vi "generateSQL.vi"(0 "input cluster":T1) -> (1 "SQL command (mote)":string, 2 "SQL command (plc)":string, 3 "SQL command (counter and manual)":string)   [LabVIEW 2011]
panel:
  out "plc":string[](array[string])
  out "mote":string[](array[string])
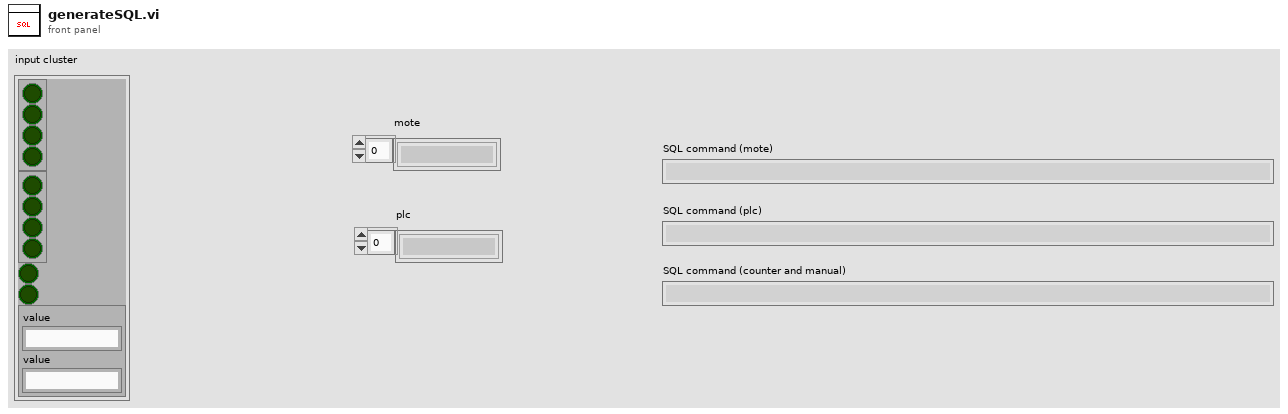
[diagram p1: front panel]
types:
  T1 = cluster{cluster{bool, bool, bool, bool}, cluster{bool, bool, bool, bool}, bool, bool, cluster{"value":string, "value":string}}
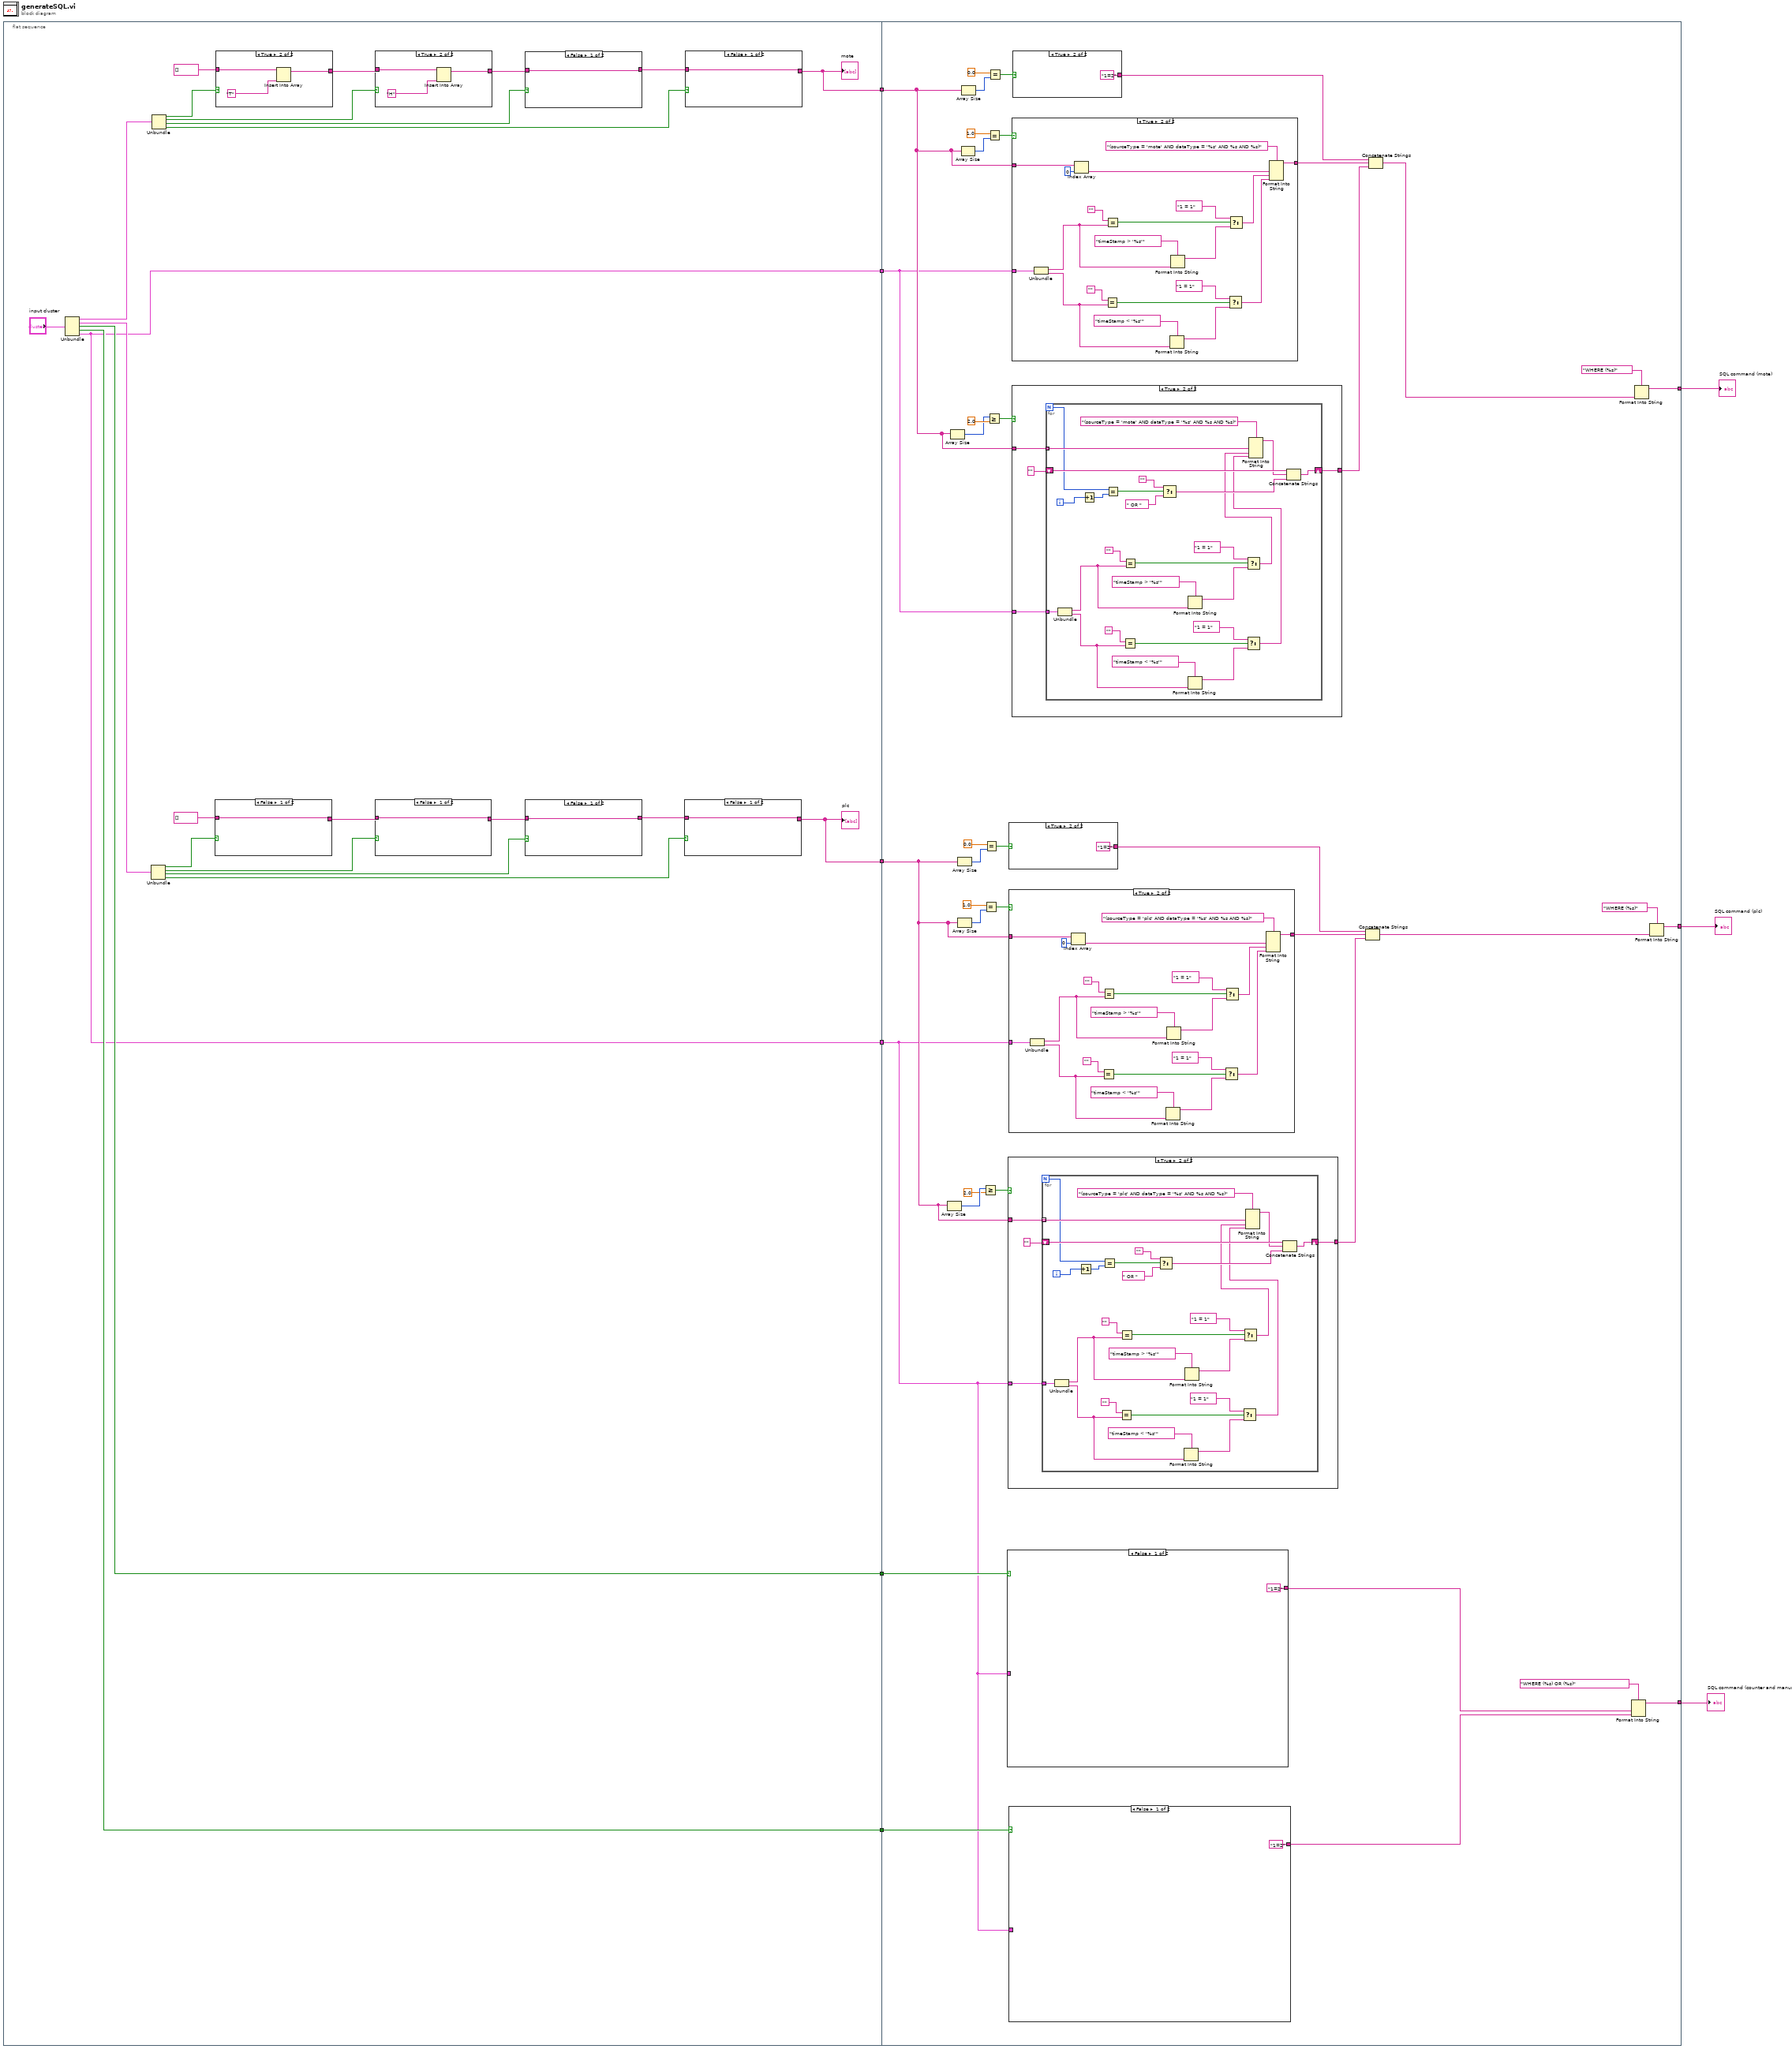
[diagram p0: block diagram]
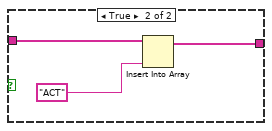
[diagram p2: hidden frame]
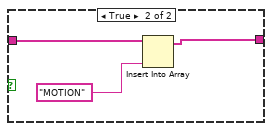
[diagram p3: hidden frame]
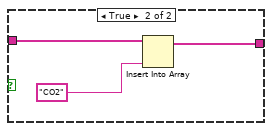
[diagram p4: hidden frame]
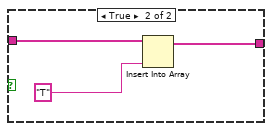
[diagram p5: hidden frame]
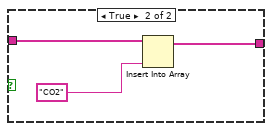
[diagram p6: hidden frame]
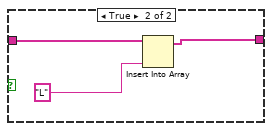
[diagram p7: hidden frame]
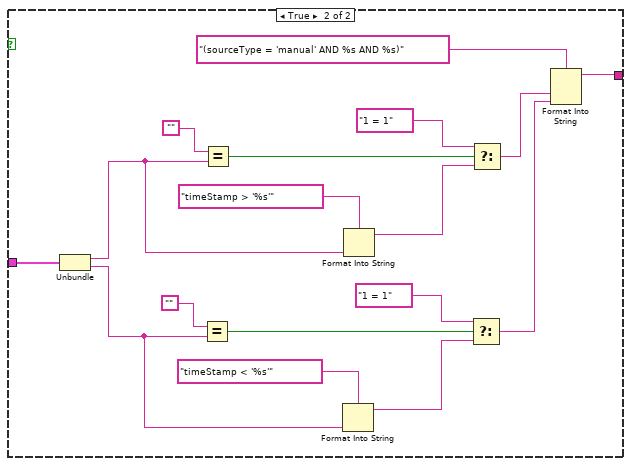
[diagram p10: hidden frame]
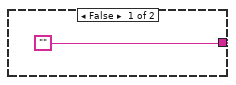
[diagram p11: hidden frame]
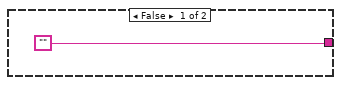
[diagram p12: hidden frame]
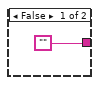
[diagram p13: hidden frame]
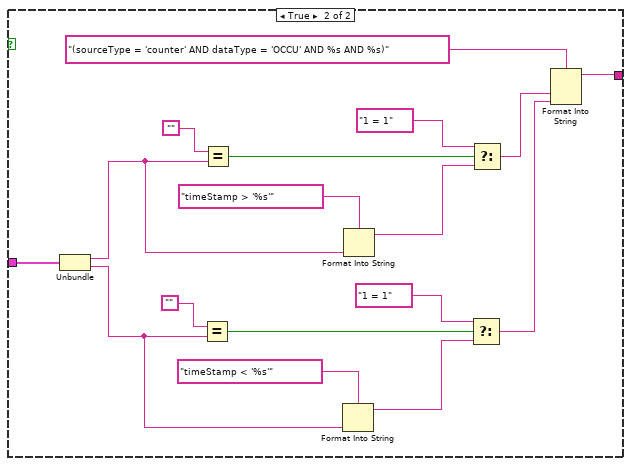
[diagram p14: hidden frame]
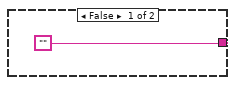
[diagram p15: hidden frame]
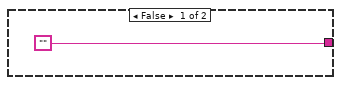
[diagram p16: hidden frame]
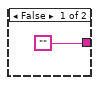
[diagram p17: hidden frame]
diagram:
  n1 = flat-sequence {
    tunnel: [w14] -> w9
    tunnel: [w13] -> w7
    tunnel: [w12] -> w6
    tunnel: [w10] -> w5
    tunnel: [w11] -> w4
    tunnel: [w10] -> w3
    tunnel: w9 -> [w93]
    tunnel: [w90] -> w8
    tunnel: w7 -> [w89]
    tunnel: w6 -> [w74]
    tunnel: w5 -> [w88]
    tunnel: w4 -> [w75]
    tunnel: w3 -> [w73]
    tunnel: [w69] -> w2
    tunnel: [w68] -> w1
    frame #0 {
      n2 = Unbundle("input cluster") -> (w32:cluster{bool, bool, bool, bool}, w31:cluster{bool, bool, bool, bool}, w13:bool, w12:bool, w10:cluster{"value":string, "value":string})
      n3 = Unbundle(w31) -> (w18:bool, w17:bool, w16:bool, w15:bool)
      n4 = Unbundle(w32) -> (w30:bool, w28:bool, w26:bool, w25:bool)
      n5 = case shown="False" w18 {
        tunnel: string[] [] -> [w46 w48]
        tunnel: [w46 w47] -> w20
        frame False {
        }
        frame True {
          n6 = Insert Into Array(array=w48, new element="T") -> (w47:string[])  [unwired: 1 in]
        }
      }
      n7 = case shown="True" w30 {
        tunnel: string[] [] -> [w62 w64]
        tunnel: [w62 w63] -> w27
        frame False {
        }
        frame True {
          n8 = Insert Into Array(array=w64, new element="T") -> (w63:string[])  [unwired: 1 in]
        }
      }
      n9 = case shown="False" w17 {
        tunnel: w20 -> [w42 w44]
        tunnel: [w42 w43] -> w21
        frame False {
        }
        frame True {
          n10 = Insert Into Array(array=w44, new element="CO2") -> (w43:string[])  [unwired: 1 in]
        }
      }
      n11 = case shown="True" w28 {
        tunnel: w27 -> [w58 w60]
        tunnel: [w58 w59] -> w24
        frame False {
        }
        frame True {
          n12 = Insert Into Array(array=w60, new element="H") -> (w59:string[])  [unwired: 1 in]
        }
      }
      n13 = case shown="False" w16 {
        tunnel: w21 -> [w38 w40]
        tunnel: [w38 w39] -> w22
        frame False {
        }
        frame True {
          n14 = Insert Into Array(array=w40, new element="MOTION") -> (w39:string[])  [unwired: 1 in]
        }
      }
      n15 = case shown="False" w26 {
        tunnel: w24 -> [w54 w56]
        tunnel: [w54 w55] -> w23
        frame False {
        }
        frame True {
          n16 = Insert Into Array(array=w56, new element="L") -> (w55:string[])  [unwired: 1 in]
        }
      }
      n17 = case shown="False" w15 {
        tunnel: w22 -> [w34 w36]
        tunnel: [w34 w35] -> w11
        frame False {
        }
        frame True {
          n18 = Insert Into Array(array=w36, new element="ACT") -> (w35:string[])  [unwired: 1 in]
        }
      }
      "plc" <- w11
      n19 = case shown="False" w25 {
        tunnel: w23 -> [w50 w52]
        tunnel: [w50 w51] -> w14
        frame False {
        }
        frame True {
          n20 = Insert Into Array(array=w52, new element="CO2") -> (w51:string[])  [unwired: 1 in]
        }
      }
      "mote" <- w14
    }
    frame #1 {
      n21 = Array Size(array=w75) -> (size(s)=w84:i32)
      n22 = Array Size(array=w93) -> (size(s)=w97:i32)
      n23 = Array Size(array=w75) -> (size(s)=w80:i32)
      n24 = Array Size(array=w75) -> (size(s)=w77:i32)
      n25 = Array Size(array=w93) -> (size(s)=w101:i32)
      n26 = Array Size(array=w93) -> (size(s)=w104:i32)
      n27 = Greater Or Equal?(x=w84, y=2.0) -> (x >= y?=w82:bool)
      n28 = Equal?(x=1.0, y=w80) -> (x = y?=w79:bool)
      n29 = Equal?(x=0.0, y=w77) -> (x = y?=w78:bool)
      n30 = Greater Or Equal?(x=w97, y=2.0) -> (x >= y?=w99:bool)
      n31 = Equal?(x=1.0, y=w101) -> (x = y?=w102:bool)
      n32 = Equal?(x=0.0, y=w104) -> (x = y?=w103:bool)
      n33 = case shown="False" w89 {
        tunnel: ["1=2" w180] -> w67
        tunnel: w73 -> [_ w184]
        frame False {
        }
        frame True {
          n34 = Unbundle(w184) -> ("value"=w192:string, "value"=w185:string)
          n35 = Equal?(x="", y=w185) -> (x = y?=w187:bool)
          n36 = Equal?(x="", y=w192) -> (x = y?=w195:bool)
          n37 = Format Into String(format string="timeStamp < '%s'", w185) -> (resulting string=w189:string)  [unwired: 2 in, 1 out]
          n38 = Format Into String(format string="timeStamp > '%s'", w192) -> (resulting string=w193:string)  [unwired: 2 in, 1 out]
          n39 = Select(t="1 = 1", s=w187, f=w189) -> (s? t:f=w182:string)
          n40 = Select(t="1 = 1", s=w195, f=w193) -> (s? t:f=w183:string)
          n41 = Format Into String(format string="(sourceType = 'counter' AND dataType = 'OCCU' AND %s AND %s)", w183, w182) -> (resulting string=w180:string)  [unwired: 2 in, 1 out]
        }
      }
      n42 = case shown="True" w82 {
        tunnel: w75 -> [_ w126]
        tunnel: ["" w127] -> w87
        tunnel: w73 -> [_ w125]
        frame False {
        }
        frame True {
          n43 = for {
            N -> [w150]
            shift-right: [w152] -> w127
            shift-left: "" -> [w154]
            tunnel: w126 -> [w151] mode=indexing
            tunnel: w125 -> [w129]
            i -> [w148]
            n44 = Unbundle(w129) -> ("value"=w136:string, "value"=w143:string)
            n45 = Increment(x=w148) -> (x+1=w149:i32)
            n46 = Equal?(x=w150, y=w149) -> (x = y?=w147:bool)
            n47 = Equal?(x="", y=w143) -> (x = y?=w141:bool)
            n48 = Equal?(x="", y=w136) -> (x = y?=w133:bool)
            n49 = Select(t="", s=w147, f=" OR ") -> (s? t:f=w144:string)
            n50 = Format Into String(format string="timeStamp < '%s'", w143) -> (resulting string=w139:string)  [unwired: 2 in, 1 out]
            n51 = Format Into String(format string="timeStamp > '%s'", w136) -> (resulting string=w135:string)  [unwired: 2 in, 1 out]
            n52 = Select(t="1 = 1", s=w141, f=w139) -> (s? t:f=w130:string)
            n53 = Select(t="1 = 1", s=w133, f=w135) -> (s? t:f=w131:string)
            n54 = Format Into String(format string="(sourceType = 'plc' AND dataType = '%s' AND %s AND %s)", w151, w131, w130) -> (resulting string=w153:string)  [unwired: 2 in, 1 out]
            n55 = Concatenate Strings(w154, w153, w144) -> (w152:string)
          }
        }
      }
      n56 = case shown="True" w79 {
        tunnel: w75 -> [_ w176]
        tunnel: ["" w172] -> w86
        tunnel: w73 -> [_ w157]
        frame False {
        }
        frame True {
          n57 = Unbundle(w157) -> ("value"=w167:string, "value"=w160:string)
          n58 = Index Array(array=w176, index=0) -> (element=w173:string)
          n59 = Equal?(x="", y=w160) -> (x = y?=w162:bool)
          n60 = Equal?(x="", y=w167) -> (x = y?=w170:bool)
          n61 = Format Into String(format string="timeStamp < '%s'", w160) -> (resulting string=w164:string)  [unwired: 2 in, 1 out]
          n62 = Format Into String(format string="timeStamp > '%s'", w167) -> (resulting string=w168:string)  [unwired: 2 in, 1 out]
          n63 = Select(t="1 = 1", s=w162, f=w164) -> (s? t:f=w158:string)
          n64 = Select(t="1 = 1", s=w170, f=w168) -> (s? t:f=w159:string)
          n65 = Format Into String(format string="(sourceType = 'plc' AND dataType = '%s' AND %s AND %s)", w173, w159, w158) -> (resulting string=w172:string)  [unwired: 2 in, 1 out]
        }
      }
      n66 = case shown="True" w78 {
        tunnel: ["" "1=2"] -> w85
        frame False {
        }
        frame True {
        }
      }
      n67 = case shown="False" w74 {
        tunnel: ["1=2" w107] -> w66
        tunnel: w73 -> [_ w111]
        frame False {
        }
        frame True {
          n68 = Unbundle(w111) -> ("value"=w119:string, "value"=w112:string)
          n69 = Equal?(x="", y=w112) -> (x = y?=w114:bool)
          n70 = Equal?(x="", y=w119) -> (x = y?=w122:bool)
          n71 = Format Into String(format string="timeStamp < '%s'", w112) -> (resulting string=w116:string)  [unwired: 2 in, 1 out]
          n72 = Format Into String(format string="timeStamp > '%s'", w119) -> (resulting string=w120:string)  [unwired: 2 in, 1 out]
          n73 = Select(t="1 = 1", s=w114, f=w116) -> (s? t:f=w109:string)
          n74 = Select(t="1 = 1", s=w122, f=w120) -> (s? t:f=w110:string)
          n75 = Format Into String(format string="(sourceType = 'manual' AND %s AND %s)", w110, w109) -> (resulting string=w107:string)  [unwired: 2 in, 1 out]
        }
      }
      n76 = case shown="True" w99 {
        tunnel: w93 -> [_ w199]
        tunnel: ["" w200] -> w94
        tunnel: w88 -> [_ w198]
        frame False {
        }
        frame True {
          n77 = for {
            N -> [w223]
            shift-right: [w225] -> w200
            shift-left: "" -> [w227]
            tunnel: w199 -> [w224] mode=indexing
            tunnel: w198 -> [w202]
            i -> [w221]
            n78 = Unbundle(w202) -> ("value"=w209:string, "value"=w216:string)
            n79 = Increment(x=w221) -> (x+1=w222:i32)
            n80 = Equal?(x=w223, y=w222) -> (x = y?=w220:bool)
            n81 = Equal?(x="", y=w216) -> (x = y?=w214:bool)
            n82 = Equal?(x="", y=w209) -> (x = y?=w206:bool)
            n83 = Select(t="", s=w220, f=" OR ") -> (s? t:f=w217:string)
            n84 = Format Into String(format string="timeStamp < '%s'", w216) -> (resulting string=w212:string)  [unwired: 2 in, 1 out]
            n85 = Format Into String(format string="timeStamp > '%s'", w209) -> (resulting string=w208:string)  [unwired: 2 in, 1 out]
            n86 = Select(t="1 = 1", s=w214, f=w212) -> (s? t:f=w203:string)
            n87 = Select(t="1 = 1", s=w206, f=w208) -> (s? t:f=w204:string)
            n88 = Format Into String(format string="(sourceType = 'mote' AND dataType = '%s' AND %s AND %s)", w224, w204, w203) -> (resulting string=w226:string)  [unwired: 2 in, 1 out]
            n89 = Concatenate Strings(w227, w226, w217) -> (w225:string)
          }
        }
      }
      n90 = case shown="True" w102 {
        tunnel: w93 -> [_ w249]
        tunnel: ["" w245] -> w95
        tunnel: w88 -> [_ w230]
        frame False {
        }
        frame True {
          n91 = Unbundle(w230) -> ("value"=w240:string, "value"=w233:string)
          n92 = Index Array(array=w249, index=0) -> (element=w246:string)
          n93 = Equal?(x="", y=w233) -> (x = y?=w235:bool)
          n94 = Equal?(x="", y=w240) -> (x = y?=w243:bool)
          n95 = Format Into String(format string="timeStamp < '%s'", w233) -> (resulting string=w237:string)  [unwired: 2 in, 1 out]
          n96 = Format Into String(format string="timeStamp > '%s'", w240) -> (resulting string=w241:string)  [unwired: 2 in, 1 out]
          n97 = Select(t="1 = 1", s=w235, f=w237) -> (s? t:f=w231:string)
          n98 = Select(t="1 = 1", s=w243, f=w241) -> (s? t:f=w232:string)
          n99 = Format Into String(format string="(sourceType = 'mote' AND dataType = '%s' AND %s AND %s)", w246, w232, w231) -> (resulting string=w245:string)  [unwired: 2 in, 1 out]
        }
      }
      n100 = case shown="True" w103 {
        tunnel: ["" "1=2"] -> w96
        frame False {
        }
        frame True {
        }
      }
      n101 = Concatenate Strings(w85, w86, w87) -> (w70:string)
      n102 = Concatenate Strings(w96, w95, w94) -> (w91:string)
      n103 = Format Into String(format string="WHERE (%s) OR (%s)", w67, w66) -> (resulting string=w68:string)  [unwired: 2 in, 1 out]
      n104 = Format Into String(format string="WHERE (%s)", w91) -> (resulting string=w90:string)  [unwired: 2 in, 1 out]
      n105 = Format Into String(format string="WHERE (%s)", w70) -> (resulting string=w69:string)  [unwired: 2 in, 1 out]
    }
  }
  "SQL command (mote)" <- w8
  "SQL command (plc)" <- w2
  "SQL command (counter and manual)" <- w1
